vi "DeCoF truncate history.vi"(3 "remember cursor in":i32, 4 "maximum length":i32=65535, 5 "history in":string) -> (0 "remember cursor out":i32, 2 "history out":string)   [LabVIEW 2013]
doc: "This VI truncates the content of the terminal history if it exceeds the given maximum number of characters."
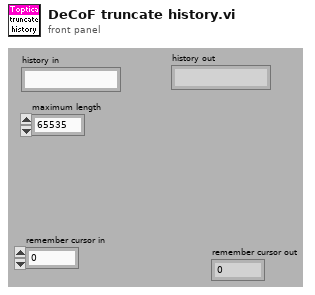
[diagram p1: front panel]
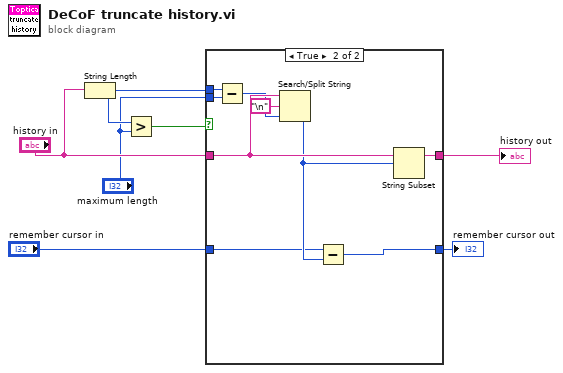
[diagram p0: block diagram]
diagram:
  n1 = String Length(string="history in") -> (length=w4:i32)
  n2 = Greater?(x=w4, y="maximum length") -> (0:w5:bool)
  n3 = case shown="True" w5 {
    tunnel: [w9 w18] -> w7
    tunnel: "history in" -> [w9 w16]
    tunnel: w4 -> [_ w13]
    tunnel: "maximum length" -> [_ w17]
    tunnel: "remember cursor in" -> [w8 w11]
    tunnel: [w8 w10] -> w1
    frame False {
    }
    frame True {
      n4 = Subtract(x=w13, y=w17) -> (x-y=w15:i32)
      n5 = Search/Split String(string=w16, search string/char (-)="\n", offset (0)=w15) -> (offset of match=w12:i32)  [unwired: 2 out]
      n6 = Subtract(x=w11, y=w12) -> (x-y=w10:i32)
      n7 = String Subset(string=w16, offset (0)=w12) -> (substring=w18:string)  [unwired: 1 in]
    }
  }
  "history out" <- w7
  "remember cursor out" <- w1
